vi "save_config_file.vi"(8 "error in (no error)":errorcluster, 9 "config cluster variant":variant, 11 "ExperimentControllerDL090130Interval in":refnum<class "ExperimentControllerDL090130Interval.lvclass">) -> (0 "error out":errorcluster, 3 "ExperimentControllerDL090130Interval out":refnum<class "ExperimentControllerDL090130Interval.lvclass">)   [LabVIEW 2010]
uses:
  ExperimentControllerDL090130Interval.lvclass
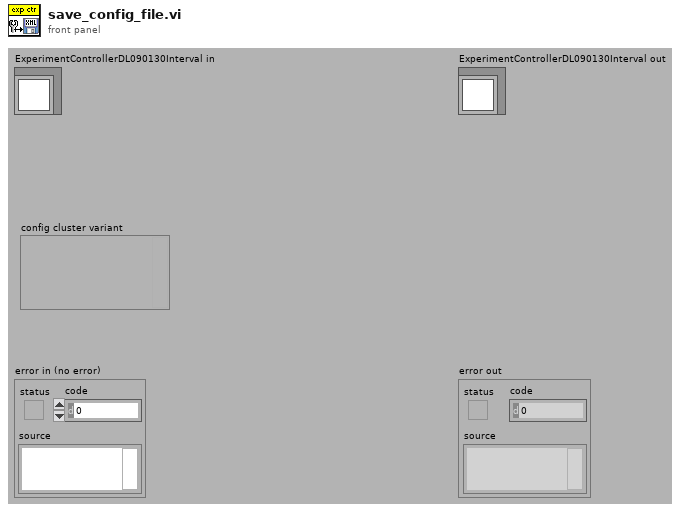
[diagram p1: front panel]
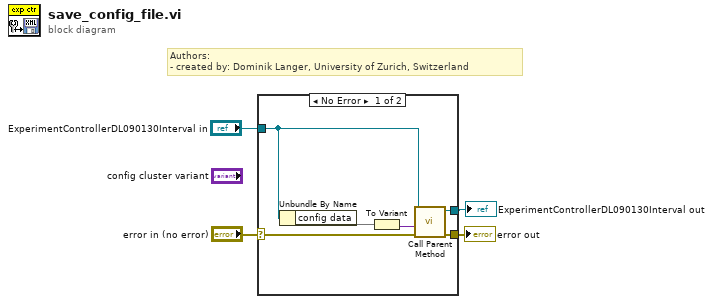
[diagram p0: block diagram]
diagram:
  # "Authors: \n- created by: Dominik Langer, University of Zurich, Switzerland"
  n1 = case shown="No Error" "error in (no error)" {
    selector: "error in (no error)" -> [w8 w11]
    tunnel: [w10 w11] -> w4
    tunnel: [w9 w12] -> w3
    tunnel: "ExperimentControllerDL090130Interval in" -> [w5 w12]
    frame No Error {
      n2 = Unbundle By Name(w5) -> ("config data"=w6)
      n3 = To Variant(anything=w6) -> (Variant=w7:variant)
      n4 = call-parent "Call Parent Method"("error in (no error)"=w8, "config cluster variant"=w7, "GenericPlugin in"=w5) -> ("error out"=w10:errorcluster, "GenericPlugin out"=w9:refnum<class "ExperimentControllerDL090130Interval.lvclass">)  [unwired: 7 in]
    }
    frame Error {
    }
  }
  "error out" <- w4
  "ExperimentControllerDL090130Interval out" <- w3
